vi "rs3 get library path.vi"() -> (0 "Realsense 2 Library Path":path)   [LabVIEW 2017, in "libRealSense3.lvlib"]
uses:
  libRealSense3.lvlib
  <vilib>/Utility/sysdir.llb/System Directory Type.ctl
panel:
  out "file or folder exists?":bool
  # "RS3 Get Library Path"
  # "(C) Intel Corp. 2017,  AGJ"
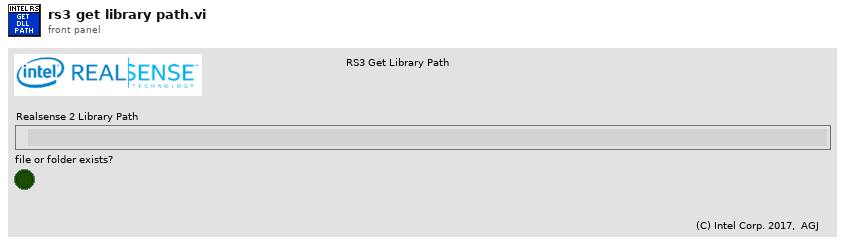
[diagram p1: front panel]
types:
  T1 = typedef "System Directory Type.ctl" = i32
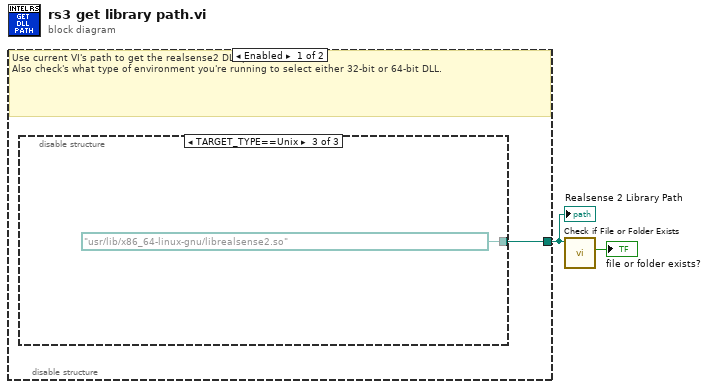
[diagram p0: block diagram]
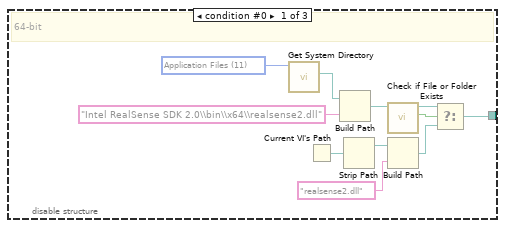
[diagram p2: hidden frame]
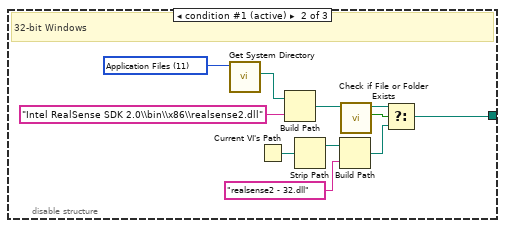
[diagram p3: hidden frame]
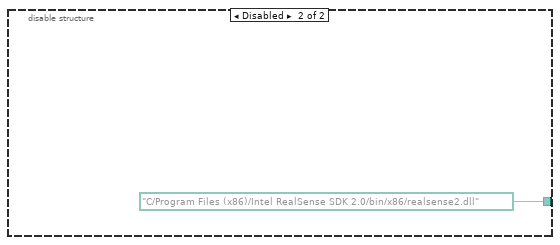
[diagram p4: hidden frame]
diagram:
  n1 = disable-structure shown="Enabled" {
    disable-tunnel: [w3 path "C:/Program Files (x86)/Intel RealSense SDK 2.0/bin/x86/realsense2.dll"] -> w2
    frame Enabled {
      # "Use current VI's path to get the realsense2 DLL path.\nAlso check's what type of environment you're running to select either 32-bit or 64-bit DLL."
      n2 = disable-structure shown="TARGET_TYPE==Unix" {
        disable-tunnel: [w4 w15 path "/usr/lib/x86_64-linux-gnu/librealsense2.so"] -> w3
        frame condition #0 {
          w6 = T1 11 items=["User Home"=0, "User Desktop"=1, "User Documents"=2, "User Application Data"=3, "User Preferences"=4, "User Temporary"=5, "Public Documents"=6, "Public Application Data"=7, "Public Preferences"=8, "Public Cache"=13, "System Core Libraries"=9, "System Installed Libraries"=10, "Application Files"=11, "Boot Volume Root"=12] ("system directory type")
          # "64-bit"
          n3 = call <vilib>:"Get System Directory.vi"("system directory type"=w6) -> ("system directory"=w8:path)  [unwired: 10 in]
          n4 = Current VI's Path() -> (path=w10:path)
          n5 = Build Path(base path=w8, name or relative path="Intel RealSense SDK 2.0\\bin\\x64\\realsense2.dll") -> (appended path=w5:path)
          n6 = Strip Path(path=w10) -> (stripped path=w11:path)  [unwired: 1 out]
          n7 = call <vilib>:"Check if File or Folder Exists.vi"("path"=w5) -> ("file or folder exists?"=w14:bool, "dup path"=w13:path)  [unwired: 8 in, 1 out]
          n8 = Build Path(base path=w11, name or relative path="realsense2.dll") -> (appended path=w12:path)
          n9 = Select(t=w13, s=w14, f=w12) -> (s? t:f=w4:path)
        }
        frame condition #1 (active) {
          w17 = T1 11 items=["User Home"=0, "User Desktop"=1, "User Documents"=2, "User Application Data"=3, "User Preferences"=4, "User Temporary"=5, "Public Documents"=6, "Public Application Data"=7, "Public Preferences"=8, "Public Cache"=13, "System Core Libraries"=9, "System Installed Libraries"=10, "Application Files"=11, "Boot Volume Root"=12] ("system directory type")
          # "32-bit Windows"
          n10 = call <vilib>:"Get System Directory.vi"("system directory type"=w17) -> ("system directory"=w19:path)  [unwired: 10 in]
          n11 = Current VI's Path() -> (path=w23:path)
          n12 = Build Path(base path=w19, name or relative path="Intel RealSense SDK 2.0\\bin\\x86\\realsense2.dll") -> (appended path=w16:path)
          n13 = Strip Path(path=w23) -> (stripped path=w24:path)  [unwired: 1 out]
          n14 = Build Path(base path=w24, name or relative path="realsense2 - 32.dll") -> (appended path=w25:path)
          n15 = call <vilib>:"Check if File or Folder Exists.vi"("path"=w16) -> ("file or folder exists?"=w22:bool, "dup path"=w21:path)  [unwired: 8 in, 1 out]
          n16 = Select(t=w21, s=w22, f=w25) -> (s? t:f=w15:path)
        }
        frame condition #2 {
        }
      }
    }
    frame Disabled {
    }
  }
  "Realsense 2 Library Path" <- w2
  n17 = call <vilib>:"Check if File or Folder Exists.vi"("path"=w2) -> ("file or folder exists?"=→"file or folder exists?":bool)  [unwired: 8 in, 2 out]
